vi "Next_Point_Step.vi"(11 "Current State":T1(ring)) -> (3 "Next State":T1(ring))   [LabVIEW 2025]
uses:
  CTLS/PointStep.ctl
panel:
  in  "PointStep.ctl In":T2={"Next State"=enum."1. Scan_1", "Current State"=enum."1. Scan_1"}
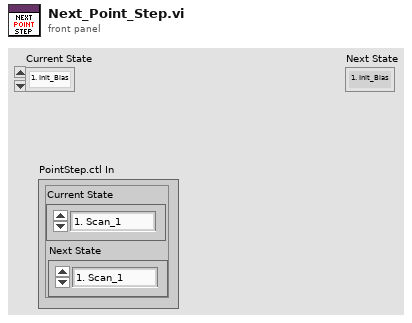
[diagram p1: front panel]
types:
  T1 = enum16{"1. Init_Bias", "2. Init_Scan", "3. Field_Stable", "4. Temp_stable", "1. Scan_1", "2. DC_SF_1", "3. DC_BS_1", "4. Bias", "5. Scan_2", "6. DC_SF_2", "7. DC_BS_2", "8. Done"}
  T2 = typedef "PointStep.ctl" = cluster{"Next State":enum16{"1. Init_Bias", "2. Init_Scan", "3. Field_Stable", "4. Temp_stable", "1. Scan_1", "2. DC_SF_1", "3. DC_BS_1", "4. Bias", "5. Scan_2", "6. DC_SF_2", "7. DC_BS_2", "8. Done"}, "Current State":enum16{"1. Init_Bias", "2. Init_Scan", "3. Field_Stable", "4. Temp_stable", "1. Scan_1", "2. DC_SF_1", "3. DC_BS_1", "4. Bias", "5. Scan_2", "6. DC_SF_2", "7. DC_BS_2", "8. Done"}}
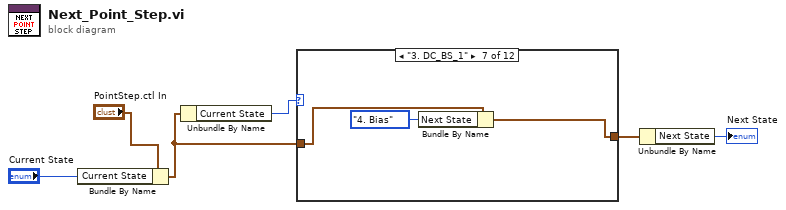
[diagram p0: block diagram]
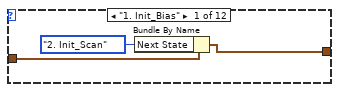
[diagram p2: hidden frame]
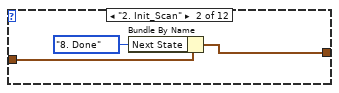
[diagram p3: hidden frame]
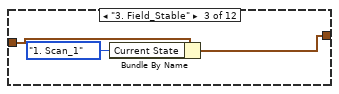
[diagram p4: hidden frame]
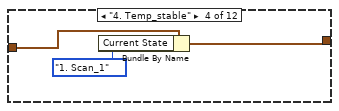
[diagram p5: hidden frame]
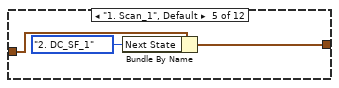
[diagram p6: hidden frame]
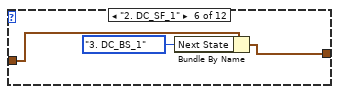
[diagram p7: hidden frame]
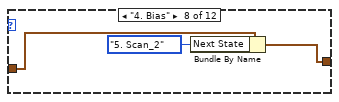
[diagram p8: hidden frame]
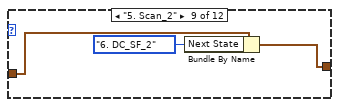
[diagram p9: hidden frame]
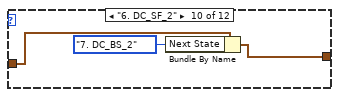
[diagram p10: hidden frame]
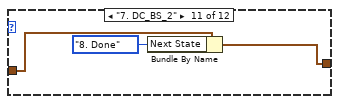
[diagram p11: hidden frame]
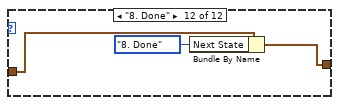
[diagram p12: hidden frame]
diagram:
  n1 = Bundle By Name(cluster="PointStep.ctl In", "Current State"="Current State") -> (w4:T2)
  n2 = Unbundle By Name(w4) -> ("Current State"=w6:T1)
  n3 = case shown="\"3. DC_BS_1\"" w6 {
    tunnel: w4 -> [w9 w12 w15 w18 w21 w24 w27 w30 w33 w36 w39 w42]
    tunnel: [w8 w11 w14 w17 w20 w23 w26 w29 w32 w35 w38 w41] -> w3
    frame "1. Init_Bias" {
      n4 = Bundle By Name(cluster=w9, "Next State"=T1."2. Init_Scan") -> (w8:T2)
    }
    frame "2. Init_Scan" {
      n5 = Bundle By Name(cluster=w12, "Next State"=T1."8. Done") -> (w11:T2)
    }
    frame "3. Field_Stable" {
      n6 = Bundle By Name(cluster=w15, "Current State"=T1."1. Scan_1") -> (w14:T2)
    }
    frame "4. Temp_stable" {
      n7 = Bundle By Name(cluster=w18, "Current State"=T1."1. Scan_1") -> (w17:T2)
    }
    frame "1. Scan_1", Default {
      n8 = Bundle By Name(cluster=w21, "Next State"=T1."2. DC_SF_1") -> (w20:T2)
    }
    frame "2. DC_SF_1" {
      n9 = Bundle By Name(cluster=w24, "Next State"=T1."3. DC_BS_1") -> (w23:T2)
    }
    frame "3. DC_BS_1" {
      n10 = Bundle By Name(cluster=w27, "Next State"=T1."4. Bias") -> (w26:T2)
    }
    frame "4. Bias" {
      n11 = Bundle By Name(cluster=w30, "Next State"=T1."5. Scan_2") -> (w29:T2)
    }
    frame "5. Scan_2" {
      n12 = Bundle By Name(cluster=w33, "Next State"=T1."6. DC_SF_2") -> (w32:T2)
    }
    frame "6. DC_SF_2" {
      n13 = Bundle By Name(cluster=w36, "Next State"=T1."7. DC_BS_2") -> (w35:T2)
    }
    frame "7. DC_BS_2" {
      n14 = Bundle By Name(cluster=w39, "Next State"=T1."8. Done") -> (w38:T2)
    }
    frame "8. Done" {
      n15 = Bundle By Name(cluster=w42, "Next State"=T1."8. Done") -> (w41:T2)
    }
  }
  n16 = Unbundle By Name(w3) -> ("Next State"=→"Next State":T1)
